vi "ZE_Recorder_TempChanelFGV.vi"(8 "error in":errorcluster, 9 "Config In":T2={"ParameterBlock"=variant, "TempChannelType"=enum."Thermocouple"}, 10 "channel name in":string="ss" caption="channel name", 11 "Action":T4) -> (0 "error out":errorcluster, 1 "found?":bool, 2 "channel config":T2={"ParameterBlock"=variant, "TempChannelType"=enum."Thermocouple"}, 3 "channel config array":T1[](array[typedef]))   [LabVIEW 2025, in "ZE_Recorder.lvlib"]
doc: "ZE_Recorder_TempChanelFGV.vi\n----------------------------------------------\nFGV containing the temperature channel configuration\n\nInputs:\n---------------------\n- error in : Cluster; \n- Action : Enum U16; \n- Config In : Cluster; \n- channel name : String; \n\nOutputs:\n---------------------\n- error out : Cluster; \n- channel names : 1DArrayOfString; \n- channel config : Cluster; \n- found? : Boolean; \n\n----------------------------------------------\n03.07.2018\nZühlke Engineering AG\nCH-8952 Schlieren\nwww.zuehlke.com"
uses:
  ZE_Recorder.lvlib
  ZE_Recorder_TempChannelAction.ctl
  ZE_Recorder_TempParam.ctl
  ZE_Recorder_TempType.ctl
  ZE_Recorder_TempConfigCluster.ctl
panel:
  # "Connector Pane"
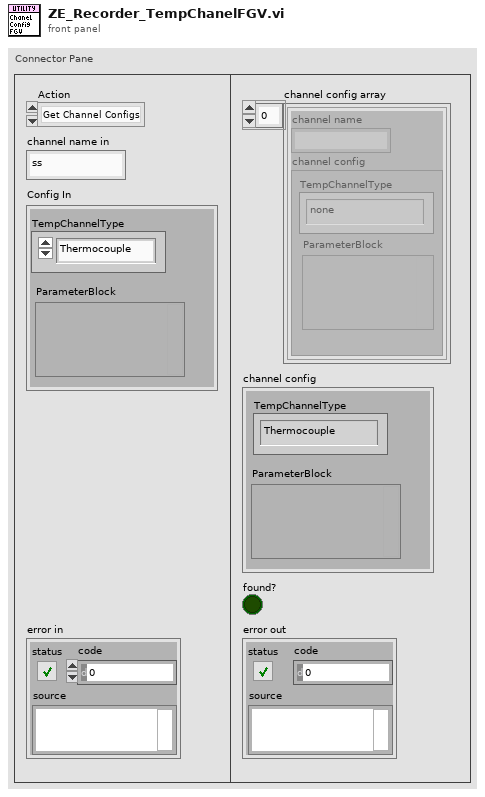
[diagram p1: front panel]
types:
  T1 = typedef "ZE_Recorder.lvlib/ZE_Recorder_TempConfigCluster.ctl" = cluster{"channel name":string, "channel config":T2}
  T2 = typedef "ZE_Recorder.lvlib/ZE_Recorder_TempParam.ctl" = cluster{"ParameterBlock":variant, "TempChannelType":T3}
  T3 = typedef "ZE_Recorder.lvlib/ZE_Recorder_TempType.ctl" = enum16{"none", "Thermocouple", "RTD", "Thermistor VE", "Thermistor CE"}
  T4 = typedef "ZE_Recorder.lvlib/ZE_Recorder_TempChannelAction.ctl" = enum16{"Get Channel Configs", "Read Config", "Add Config", "Clear"}
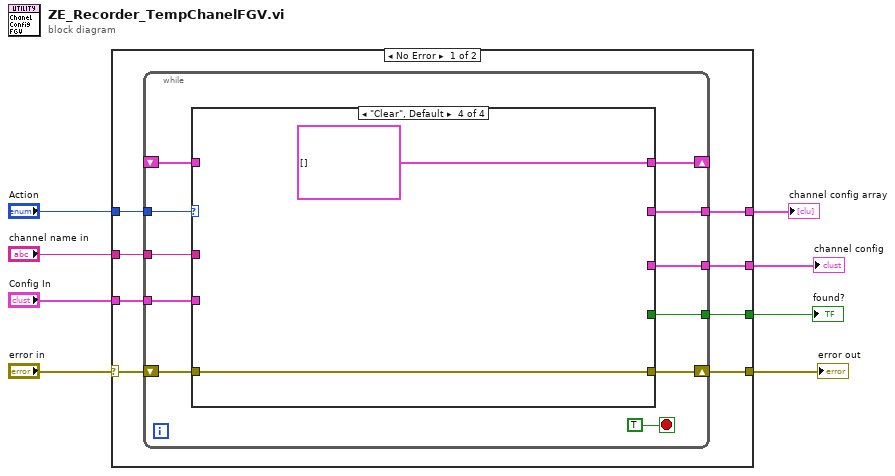
[diagram p0: block diagram]
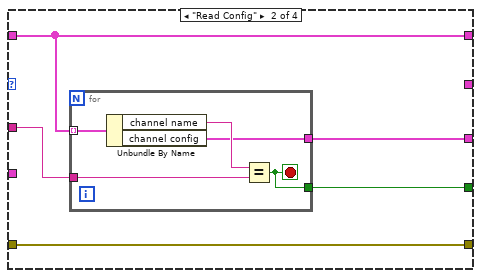
[diagram p3: hidden frame]
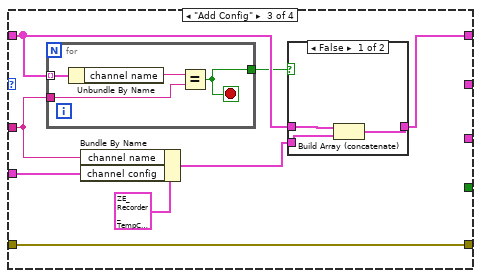
[diagram p4: hidden frame]
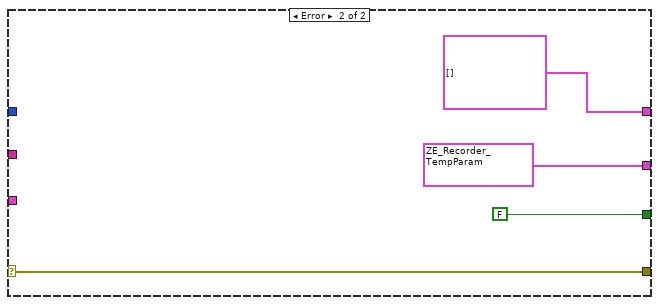
[diagram p6: hidden frame]
diagram:
  n1 = case shown="No Error" "error in" {
    selector: "error in" -> [w16 w61]
    tunnel: [w15 w61] -> w7
    tunnel: "Action" -> [w14 _]
    tunnel: "channel name in" -> [w13 _]
    tunnel: "Config In" -> [w12 _]
    tunnel: [w11 T1[] []] -> w3
    tunnel: [w10 T2 {"ParameterBlock"=variant, "TempChannelType"=enum."Thermocouple"} ("channel config")] -> w2
    tunnel: [w9 FALSE] -> w1
    frame No Error {
      n2 = while {
        shift-right: [w20] -> w15
        shift-left: w16 -> [w21]
        tunnel: w14 -> [w26]
        tunnel: w13 -> [w25]
        tunnel: w12 -> [w24]
        shift-right: [w23] -> _
        shift-left: _ -> [w22]
        tunnel: [w19] -> w11
        tunnel: [w18] -> w10
        tunnel: [w17] -> w9
        stop <- TRUE stop-if-true
        n3 = case shown="\"Clear\", Default" w26 {
          tunnel: w25 -> [_ w33 w41 _]
          tunnel: w24 -> [_ _ w46 _]
          tunnel: [w28 w34 w44 T1[] []] -> w23
          tunnel: w22 -> [w28 w34 w42 _]
          tunnel: [w29 w31 w43 w56] -> w20
          tunnel: w21 -> [w29 w31 w43 w56]
          tunnel: [w28 _ _ _] -> w19
          tunnel: [_ w32 _ _] -> w18
          tunnel: [_ w30 _ _] -> w17
          frame "Get Channel Configs" {
          }
          frame "Read Config" {
            n4 = for {
              tunnel: w34 -> [w39] mode=indexing
              tunnel: w33 -> [w37]
              tunnel: [w36] -> w32
              tunnel: [w35] -> w30
              stop <- w35 stop-if-true
              n5 = Unbundle By Name(w39) -> ("channel name"=w38:string, "channel config"=w36:T2)
              n6 = Equal?(x=w38, y=w37) -> (x = y?=w35:bool)
            }
          }
          frame "Add Config" {
            n7 = for {
              tunnel: w42 -> [w55] mode=indexing
              tunnel: w41 -> [w53]
              tunnel: [w52] -> w40
              stop <- w52 stop-if-true
              n8 = Unbundle By Name(w55) -> ("channel name"=w54:string)
              n9 = Equal?(x=w54, y=w53) -> (x = y?=w52:bool)
            }
            n10 = Bundle By Name(cluster=T1 {"channel name"="ss", "channel config"={"ParameterBlock"=variant, "TempChannelType"=enum."Thermocouple"}}, "channel name"=w41, "channel config"=w46) -> (w45:T1)
            n11 = case shown="False" w40 {
              tunnel: w45 -> [w50 _]
              tunnel: [w49 w51] -> w44
              tunnel: w42 -> [w48 w51]
              frame False {
                n12 = Build Array (concatenate)(w48, w50) -> (w49:T1[])
              }
              frame True {
              }
            }
          }
          frame "Clear", Default {
          }
        }
      }
    }
    frame Error {
    }
  }
  "error out" <- w7
  "channel config" <- w2
  "found?" <- w1
  "channel config array" <- w3
